vi "Read Lock-In Channel.vi"(7 "index":i32, 8 "error in":errorcluster, 11 "host in":refnum<class "LIA Host Interface FPGA.lvclass">) -> (0 "error out":errorcluster, 2 "unscaled data":i64[][](array[numeric]), 3 "host out":refnum<class "LIA Host Interface FPGA.lvclass">)   [LabVIEW 2018, in "LIA Host Interface FPGA.lvclass"]
uses:
  LIA Host Interface FPGA.lvclass
  Properties/FpgaSession_GET.vi
  host/Lock-In Amplifier Example Host.lvlib
  <instrlib>/_niInstr/Streaming/v1/Host/niInstr Streaming v1 Host.lvlib
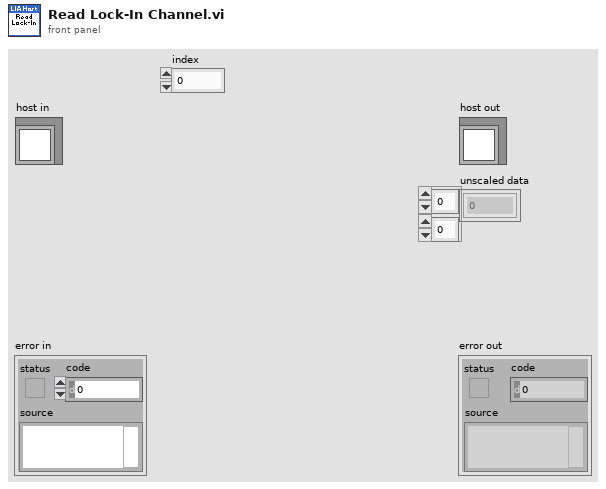
[diagram p1: front panel]
types:
  T1 = typedef "niInstr Streaming v1 Common.lvlib/Stream State.ctl" = enum8{"Idle", "Finite Transfer", "Continuous", "Done", "Error", "Not Ready", "Cancel"}
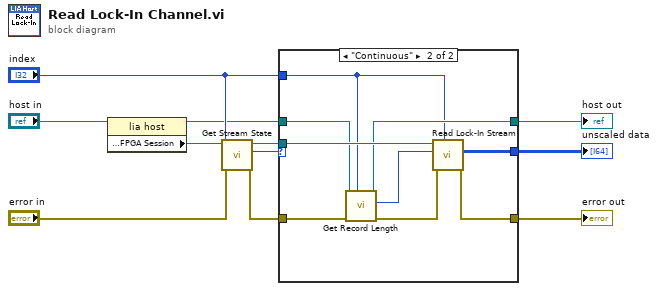
[diagram p0: block diagram]
diagram:
  n1 = property class="lia host"(reference="host in") -> (reference out=w2:refnum<class "LIA Host Interface FPGA.lvclass">, "Properties:FPGA Session"=w7:refnum<k20>)  [unwired: 1 in, 1 out]
  n2 = call <instrlib>:"Get Stream State.vi"("error in (no error)"="error in", "stream index"="index", "refnum in"=w7) -> ("error out"=w5:errorcluster, "stream state"=w4:T1, "refnum out"=w8:refnum<k20>)  [unwired: 6 in]
  n3 = case shown="\"Continuous\"" w4 {
    tunnel: [w12 w22] -> w10
    tunnel: "index" -> [_ w14]
    tunnel: w8 -> [_ w21]
    tunnel: w5 -> [w12 w18]
    tunnel: [w13 w15] -> w3
    tunnel: w2 -> [w13 w16]
    tunnel: [_ w20] -> w1
    frame Default {
    }
    frame "Continuous" {
      n4 = call "Get Record Length.vi"("instance"=w14, "error in"=w18, "lia host in"=w16) -> ("error out"=w17:errorcluster, "record length"=w19:u32, "lia host out"=w15:refnum<class "LIA Host Interface FPGA.lvclass">)  [unwired: 6 in]
      n5 = call "Read Lock-In Stream.vi"("index"=w14, "error in"=w17, "elements"=w19, "fpga session in"=w21) -> ("error out"=w22:errorcluster, "unscaled data"=w20:i64[][])  [unwired: 4 in, 2 out]
    }
  }
  "error out" <- w10
  "host out" <- w3
  "unscaled data" <- w1
